vi "SCPI.Receive.vi"(8 "error in (no error)":errorcluster, 10 "SCPI command":string, 11 "Instrument.SCPI in":refnum<class "Instrument.SCPI.lvclass">) -> (0 "error out":errorcluster, 2 "SCPI Response":string, 3 "Instrument.SCPI out":refnum<class "Instrument.SCPI.lvclass">)   [LabVIEW 2019, in "Instrument.SCPI.lvclass"]
uses:
  Instrument.SCPI.lvclass
  Typedefs/SCPI.Commands--Enum.ctl
  01597b25-3821-4342-a3c7-633ae7c306d6.vi
  01597b25-3821-4342-a3c7-633ae7c306d6.vi/269e062e-1db1-421b-ac06-1821b5ed3446.vi
  01597b25-3821-4342-a3c7-633ae7c306d6.vi/40d951c2-a9ce-4d49-b8f4-bdb62821cce5.vi
  <vilib>/Utility/Data Type/Get Type Information.vi
  <vilib>/JDP Science/JSONtext/JSON text to Variant.vi
  <vilib>/JDP Science/JSONtext/LVClass Serializer/JSONtext LVClass Serializer.lvclass
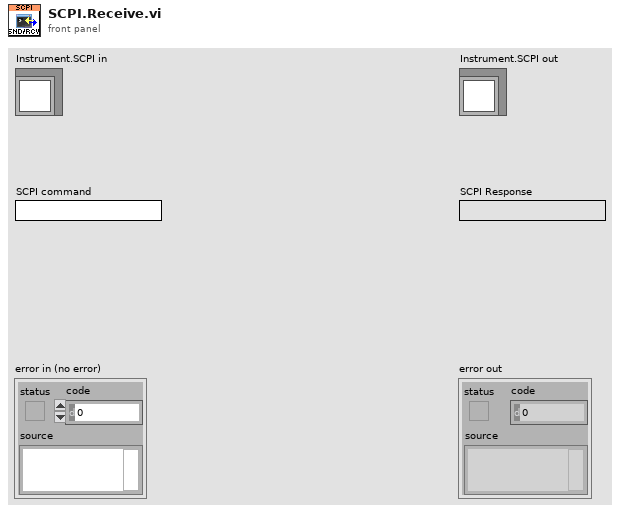
[diagram p1: front panel]
types:
  T1 = typedef "Instrument.SCPI.lvclass/SCPI.Commands--Enum.ctl" = enum16{"sendSCPI", "receiveSCPI"}
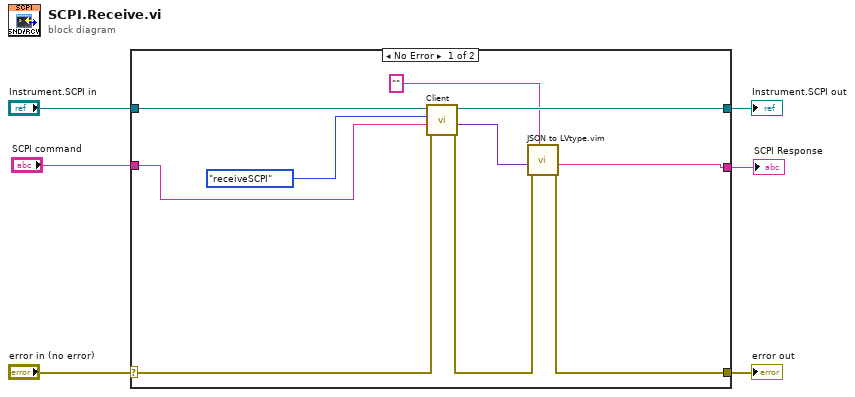
[diagram p0: block diagram]
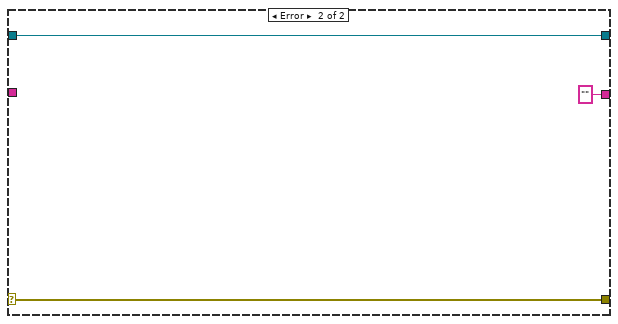
[diagram p2: hidden frame]
diagram:
  n1 = case shown="No Error" "error in (no error)" {
    selector: "error in (no error)" -> [w12 w19]
    tunnel: [w8 w19] -> w5
    tunnel: [w13 w18] -> w3
    tunnel: "Instrument.SCPI in" -> [w15 w18]
    tunnel: "SCPI command" -> [w14 _]
    tunnel: [w7 "" ("Data out")] -> w1
    frame No Error {
      n2 = call-dynamic "Client.vi"("error in (no error)"=w12, "Data in"=w14, "Command in"=SCPI.Commands--Enum."receiveSCPI" ("Commands"), "Instrument in"=w15) -> ("error out"=w9:errorcluster, "Data out"=w10:variant, "Instrument out"=w13:refnum<class "Instrument.SCPI.lvclass">)  [unwired: 4 in, 1 out]
      n3 = call "JSON to LVtype.vim"("type"="", "error in (no error)"=w9, "JSON Data in"=w10) -> ("error out"=w8:errorcluster, "Data out"=w7:string)  [unwired: 7 in]
    }
    frame Error {
    }
  }
  "error out" <- w5
  "Instrument.SCPI out" <- w3
  "SCPI Response" <- w1
